vi "Test MQTT-3.1.3-11.vi"(8 "error in (no error)":errorcluster) -> (0 "error out":errorcluster)   [LabVIEW 2013]
uses:
  source/Control Packets/CONNECT/ConnectFlags -- cluster.ctl
  <vilib>/addons/_JKI Toolkits/Caraya/classes/Assert/Assert Equal Value_Variant.vi
  source/Control Packets/CONNECT/CONNECT.lvclass
  <vilib>/addons/_JKI Toolkits/Caraya/classes/Test/Test.lvclass
  source/Control Packets/ControlPacket/ControlPacket.lvclass
  <vilib>/addons/_JKI Toolkits/Caraya/classes/Assert/Assert.lvclass
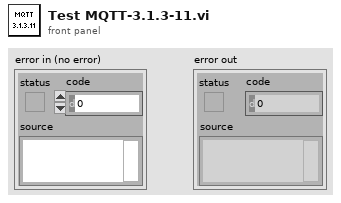
[diagram p1: front panel]
types:
  T1 = cluster{"Will Topic":string, "Will Message":string, "Username":string, "Password":string}
  T2 = typedef "CONNECT.lvclass/ConnectFlags -- cluster.ctl" = cluster{"Reserved":bool, "Clean Session":bool, "Will Flag":bool, "Will QoS 1":bool, "Will QoS 2":bool, "Will Retain":bool, "Password Flag":bool, "User Name Flag":bool}
  T3 = typedef "CONNECT.lvclass/ConnectPayload -- cluster.ctl" = cluster{"Will Topic":string, "Will Message":string, "Username":string, "Password":string}
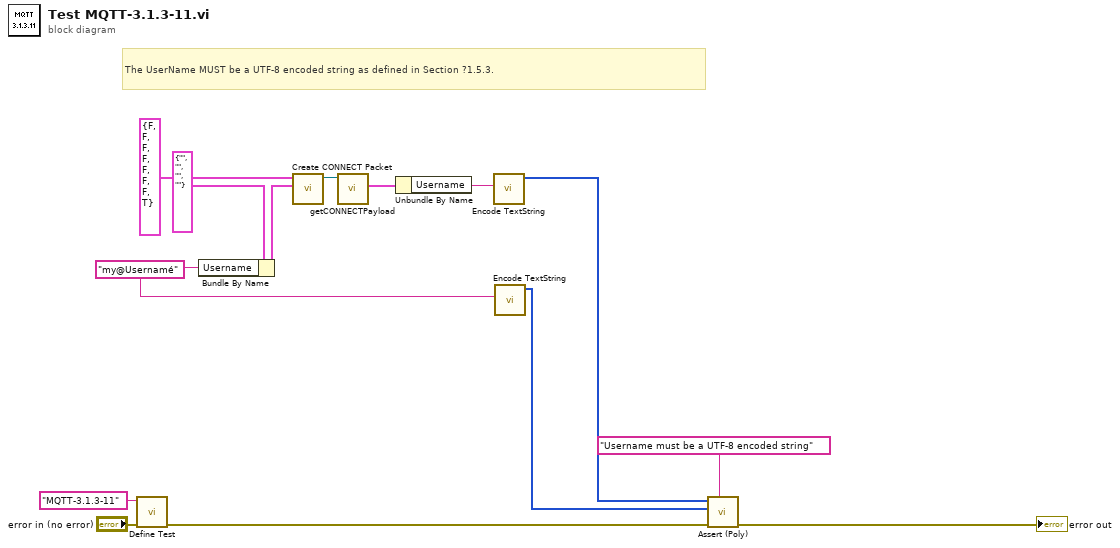
[diagram p0: block diagram]
diagram:
  w3 = "my@Usernamé" ("Username")
  # "The UserName MUST be a UTF-8 encoded string as defined in Section ?1.5.3."
  n1 = call <vilib>:"Define Test.vi"("error in (no error)"="error in (no error)", "Label (VI Title)"="MQTT-3.1.3-11") -> ("error out"=w11:errorcluster)  [unwired: 9 in]
  n2 = Bundle By Name(cluster=T1 {"Will Topic"="", "Will Message"="", "Username"="", "Password"=""} ("Payload"), "Username"=w3) -> (w5:T1)
  n3 = call "Create CONNECT Packet.vi"("Payload"=w5, "Connect Flags"=T2 {"Reserved"=FALSE, "Clean Session"=FALSE, "Will Flag"=FALSE, "Will QoS 1"=FALSE, "Will QoS 2"=FALSE, "Will Retain"=FALSE, "Password Flag"=FALSE, "User Name Flag"=TRUE}) -> ("CONNECT"=w8:refnum<class "CONNECT.lvclass">)  [unwired: 8 in, 1 out]
  n4 = call "getCONNECTPayload.vi"("CONNECT in"=w8) -> ("Payload"=w7:T3)  [unwired: 9 in, 1 out]
  n5 = Unbundle By Name(w7) -> ("Username"=w4:string)
  n6 = call "Encode TextString.vi"("Text String"=w4) -> ("Length-Prefixed Field"=w1:u8[])  [unwired: 10 in]
  n7 = call "Encode TextString.vi"("Text String"=w3) -> ("Length-Prefixed Field"=w2:u8[])  [unwired: 10 in]
  n8 = call-poly <vilib>:"Assert (Poly).vi"("Label"="Username must be a UTF-8 encoded string", "error in (no error)"=w11, "Y"=w2, "X"=w1) -> ("error out"=→"error out":errorcluster)  [unwired: 7 in]
